vi "LEMP_realtime_theory_v3.vi"() -> ()   [LabVIEW 2021]
uses:
  <vilib>/Analysis/7linalg.llb/Eigenvalue and Vectors Output Option.ctl
  <vilib>/Analysis/baseanly.llb/Matrix Type of Inverse Matrix.ctl
  <vilib>/Analysis/4window.llb/Hanning Window (DBL).vi
  <vilib>/Analysis/5stat.llb/RMS (DBL).vi
  <vilib>/Analysis/4window.llb/Hamming Window (DBL).vi
  <vilib>/Analysis/2dsp.llb/Real FFT.vi
  <vilib>/Analysis/7linalg.llb/Real Generalized Eigenvalues and Vectors.vi
  <vilib>/Analysis/7linalg.llb/Real Cholesky Factorization.vi
  <vilib>/Analysis/4window.llb/AllCosWindow (DBL).vi
  <vilib>/Analysis/baseanly.llb/Full Cholesky Factorization.vi
  <vilib>/Analysis/baseanly.llb/Full Real Matrix Cholesky Factorization.vi
  <vilib>/addons/Time Series Analysis/Series Preprocess.llb/TSA Moving Average (Array).vi
  <vilib>/Analysis/Matrix/Numeric/Conversions/Array To Matrix - RA2.vi
  <vilib>/Analysis/baseanly.llb/Real Inverse Matrix.vi
  <vilib>/Analysis/Matrix/Numeric/Multiply/Multiply - RM,RM.vi
  <vilib>/Analysis/7linalg.llb/Real Eigenvalues and Vectors.vi
  <vilib>/Analysis/Matrix/Numeric/Add/Add - RM,RM.vi
  <vilib>/gmath/statdist.llb/Normal Moments.vi
  <vilib>/gmath/NI_Gmath.lvlib
  <vilib>/Analysis/NI_AALPro.lvlib
  <vilib>/Analysis/Matrix/NI_Matrix.lvlib
  <vilib>/Analysis/NI_AALBase.lvlib
  <vilib>/DAQmx/write.llb/DAQmx Write (Digital 1D Bool NChan 1Samp 1Line).vi
  <vilib>/addons/_Advanced Signal Processing/NI_AdvSigProcTSA.lvlib
panel:
  in  "Modeling Parameters":T1
  in  "Sub Sample":bool
  out "min value":dbl=40.777955555555565
  out "max value":dbl=69.90506666666668
  in  "MASTER":bool
  in  "Tab Control":T2(tab)=enum."Check"
  out "Cycle time (ms)":dbl=0.147275536505731
  out "1st Nat. Freq. (Hz) 2":dbl=40.777955555555565 format="%#_5g"
  out "FEA Frequencies":dbl[](array[numeric])=[47.056894447356875, 51.47067845292848, 50.76081786160022]
  out "Acceleration Data":dbl[](graph) caption="Accelorometer data"
  in  "Real-Time plotting":bool
  out "Probability Density Function":cluster{i32[], dbl[]}(graph)={[9, 10, 11, 12, 13, 14, 15, 16, 17, 18, 19, 20, 21, 22, 23, 24, 25, 26], [0.09171563397251428, 0.12108231855717679, 0.143041857841436, 0.1512135165862316, 0.143041857841436, 0.12108231855717679, 0.09171563397251428, 0.062165735159412254, 0.03770542435775916, 0.020464524096401888, 0.009939041952144324, 0.004319489826678621, 0.0016798304322918924, 0.0005845793791312176, 0.00018203990329545533, 5.072648364839732e-05, 1.2648760741233286e-05, 2.8223200098705454e-06]}
  out "FFT":dbl[](graph)
  out "Frequencies":dynamicdata(graph)=[{"t0"=timestamp(0 s since 1904-01-01), "dt"=1.0, "Y"=array[322 elements]}, {"t0"=timestamp(0 s since 1904-01-01), "dt"=1.0, "Y"=array[322 elements]}]
  out "Position":dynamicdata(graph)=[{"t0"=timestamp(0 s since 1904-01-01), "dt"=1.0, "Y"=[10.0, 12.0, 10.0, 10.0, 10.0, 9.0, 10.0, 12.0, 10.0, 9.0, 9.0, 12.0, 10.0, 16.0, 11.0, 14.0, 14.0, 12.0, 12.0, 12.0, 12.0, 14.0, 14.0, 11.0, 12.0, 12.0, 12.0, 12.0, 12.0, 10.0, 12.0, 14.0, 13.0, 16.0, 14.0, 13.0, 16.0, 14.0, 11.0, 11.0, 16.0, 18.0, 11.0, 10.0, 10.0, 12.0, 10.0, 10.0, 12.0, 12.0, 10.0, 12.0, 10.0, 10.0, 10.0, 10.0, 12.0, 9.0, 11.0, 13.0, 15.0, 15.0, 16.0, 18.0, 15.0, 15.0, 17.0, 15.0, 20.0, 18.0, 15.0, 15.0, 11.0, 11.0, 11.0, 12.0, 9.0, 10.0, 10.0, 10.0, 10.0, 12.0, 14.0, 10.0, 12.0, 12.0, 10.0, 10.0, 10.0, 10.0, 10.0, 10.0, 9.0, 10.0, 12.0, 9.0, 9.0, 14.0, 11.0, 13.0, 15.0, 19.0, 19.0, 17.0, 17.0, 17.0, 21.0, 19.0, 26.0, 26.0, 26.0, 26.0, 24.0, 26.0, 24.0, 24.0, 21.0, 20.0, 20.0, 20.0, 22.0, 14.0, 16.0, 18.0, 18.0, 12.0, 10.0, 12.0, 12.0, 12.0, 16.0, 14.0, 10.0, 14.0, 16.0, 16.0, 20.0, 20.0, 22.0, 22.0, 26.0, 21.0, 19.0, 19.0, 15.0, 19.0, 19.0, 19.0, 19.0, 17.0, 20.0, 24.0, 23.0, 21.0, 21.0, 26.0, 26.0, 26.0, 26.0, 24.0, 24.0, 22.0, 20.0, 22.0, 24.0, 22.0, 24.0, 20.0, 17.0, 18.0, 16.0, 13.0, 14.0, 14.0, 12.0, 10.0, 9.0, 10.0, 11.0, 17.0, 17.0, 24.0, 21.0, 23.0, 24.0, 19.0, 21.0, 25.0, 23.0, 26.0, 25.0, 25.0, 23.0, 23.0, 21.0, 23.0, 25.0, 21.0, 26.0, 24.0, 22.0, 18.0, 14.0, 12.0, 12.0, 12.0, 10.0, 12.0, 10.0, 9.0, 10.0, 10.0, 12.0, 11.0, 10.0, 12.0, 10.0, 10.0, 10.0, 10.0, 10.0, 10.0, 10.0, 9.0, 12.0, 12.0, 11.0, 13.0, 14.0, 12.0, 12.0, 12.0, 10.0, 10.0, 12.0, 10.0, 10.0, 10.0, 9.0, 9.0, 10.0, 12.0, 12.0, 18.0, 14.0, 18.0, 15.0, 12.0, 12.0, 12.0, 14.0, 11.0, 12.0, 12.0, 12.0, 11.0, 10.0, 10.0, 9.0, 10.0, 14.0, 16.0, 12.0, 12.0, 13.0, 13.0, 15.0, 13.0, 14.0, 9.0, 9.0, 10.0, 10.0, 9.0, 10.0, 11.0, 10.0, 10.0, 12.0, 11.0, 14.0, 14.0, 12.0, 12.0, 10.0, 13.0, 15.0, 13.0, 15.0, 15.0, 21.0, 19.0, 16.0, 16.0, 14.0, 16.0, 14.0, 12.0, 10.0, 10.0, 10.0, 10.0, 14.0, 22.0, 24.0, 22.0, 26.0, 22.0, 20.0, 20.0, 19.0, 21.0, 21.0, 17.0, 19.0, 17.0, 16.0, 17.0, 14.0, 12.0, 12.0, 10.0]}, {"t0"=timestamp(0 s since 1904-01-01), "dt"=1.0, "Y"=[9.0, 9.0, 9.0, 10.0, 11.0, 11.0, 12.0, 12.0, 12.0, 12.0, 11.0, 11.0, 10.0, 10.0, 9.0, 9.0, 9.0, 9.0, 10.0, 10.0, 11.0, 11.0, 11.0, 12.0, 12.0, 13.0, 13.0, 14.0, 14.0, 14.0, 14.0, 14.0, 15.0, 15.0, 15.0, 14.0, 13.0, 13.0, 12.0, 11.0, 10.0, 10.0, 10.0, 9.0, 9.0, 9.0, 9.0, 9.0, 10.0, 11.0, 11.0, 12.0, 12.0, 13.0, 14.0, 15.0, 16.0, 16.0, 16.0, 17.0, 17.0, 17.0, 17.0, 17.0, 17.0, 17.0, 16.0, 16.0, 15.0, 15.0, 14.0, 13.0, 12.0, 11.0, 11.0, 10.0, 10.0, 10.0, 9.0, 9.0, 9.0, 9.0, 9.0, 9.0, 9.0, 10.0, 11.0, 12.0, 12.0, 13.0, 14.0, 14.0, 15.0, 15.0, 16.0, 17.0, 18.0, 19.0, 19.0, 19.0, 20.0, 20.0, 20.0, 20.0, 20.0, 19.0, 19.0, 19.0, 18.0, 18.0, 17.0, 16.0, 15.0, 15.0, 14.0, 13.0, 12.0, 11.0, 11.0, 10.0, 10.0, 10.0, 9.0, 9.0, 9.0, 9.0, 9.0, 10.0, 10.0, 11.0, 12.0, 13.0, 14.0, 15.0, 16.0, 18.0, 19.0, 20.0, 21.0, 21.0, 22.0, 22.0, 22.0, 23.0, 23.0, 23.0, 23.0, 23.0, 22.0, 22.0, 22.0, 21.0, 21.0, 20.0, 19.0, 18.0, 16.0, 15.0, 14.0, 13.0, 12.0, 12.0, 12.0, 11.0, 10.0, 10.0, 9.0, 9.0, 9.0, 9.0, 10.0, 10.0, 11.0, 12.0, 13.0, 15.0, 16.0, 18.0, 20.0, 21.0, 22.0, 23.0, 24.0, 25.0, 25.0, 25.0, 25.0, 25.0, 25.0, 25.0, 24.0, 23.0, 22.0, 21.0, 20.0, 19.0, 17.0, 15.0, 14.0, 13.0, 12.0, 11.0, 10.0, 10.0, 9.0, 9.0, 9.0, 9.0, 9.0, 9.0, 9.0, 9.0, 9.0, 9.0, 9.0, 9.0, 9.0, 10.0, 11.0, 11.0, 10.0, 9.0, 9.0, 9.0, 9.0, 9.0, 9.0, 9.0, 9.0, 9.0, 9.0, 9.0, 9.0, 9.0, 9.0, 9.0, 9.0, 9.0, 9.0, 9.0, 10.0, 13.0, 14.0, 13.0, 11.0, 10.0, 9.0, 9.0, 9.0, 9.0, 9.0, 9.0, 9.0, 9.0, 9.0, 9.0, 9.0, 9.0, 9.0, 9.0, 9.0, 10.0, 14.0, 16.0, 17.0, 14.0, 12.0, 10.0, 9.0, 9.0, 9.0, 9.0, 9.0, 9.0, 9.0, 9.0, 9.0, 9.0, 9.0, 9.0, 9.0, 9.0, 10.0, 14.0, 18.0, 19.0, 20.0, 18.0, 14.0, 10.0, 9.0, 9.0, 9.0, 9.0, 9.0, 9.0, 9.0, 9.0, 9.0, 9.0, 9.0, 9.0, 9.0, 9.0, 9.0, 10.0, 13.0, 18.0, 22.0, 22.0, 19.0, 15.0, 12.0, 10.0, 9.0, 9.0, 9.0, 9.0, 9.0, 9.0, 9.0, 9.0]}]
  in  "PDF":bool
  out "Low-Energy Warning":bool
  in  "Frequency Method":T3(ring)=enum."1-FFT-CPU"
  in  "Width":dbl=0.0508 format="%#.6f"
  in  "Density":dbl=7900.0
  in  "Height":dbl=0.00635
  in  "Length of Beam":dbl=0.3525
  in  "Young's Modulus":dbl=209500000000.0
  in  "Torsion Spring":dbl format="%#.6f"
  in  "Initial Pin node":i32
  in  "Std. Dev.":dbl=0.5 min=0.0
  in  "Eigenvalue Method":T4(ring)
  out "average cycle time (ms)":dbl=4.283940110367686 format="%0.2f"
  in  "FFT data length (data points)":i32=15000
  in  "Min. FFT Power Value (RMS)":dbl=0.02
  in  "Bound to 1st Frequency":bool=TRUE
  in  "accelerometer_mass":dbl=0.055
  in  "Std. Dev = Number of Particles / 3":bool=TRUE
  out "Std. Dev.  2":dbl=1.0
  in  "Number Of Particles":i32=3
  in  "FEA Nodes":i32=60
  in  "file name":i32
  out "FFT_data_length":i32=15000
  in  "Auto FFT length":bool
  out "Hz / per pin location":dbl=1.0
  out "FFT_frequency_resolution":dbl=1.7066666666666668
  in  "scaling_factor_Hz_per_pin_to_frequency_resolution":dbl=0.33 caption="Scale FFT Factor" format="%#_13g"
  in  "Save Acceleration Data":bool=TRUE
  in  "Mode Count":i32=3 min=1 max=10 step=1
  in  "Max Roller Velocity":dbl=3.32
  in  "Frequency selection method":T5(ring)
  in  "Use Top N freq components":i32=5 min=1 max=50 step=1
  out "Std. Dev. 2":dbl=1.0
  out "1st Nat. Freq. (Hz) 4":waveform(dbl)[](graph)=[{"t0"=timestamp(0 s since 1904-01-01), "dt"=0.004283940110367686, "Y"=array[2994 elements]}, {"t0"=timestamp(0 s since 1904-01-01), "dt"=0.004283940110367686, "Y"=array[2994 elements]}] caption="1st Nat. Freq. (Hz)"
  out "1st Nat. Freq. (Hz) 5":waveform(dbl)[](graph)=[{"t0"=timestamp(0 s since 1904-01-01), "dt"=0.004283940110367686, "Y"=array[2994 elements]}, {"t0"=timestamp(0 s since 1904-01-01), "dt"=0.004283940110367686, "Y"=array[2994 elements]}] caption="Beam Boundary condtion"
  # "Note: All Inputs are based on base SI units."
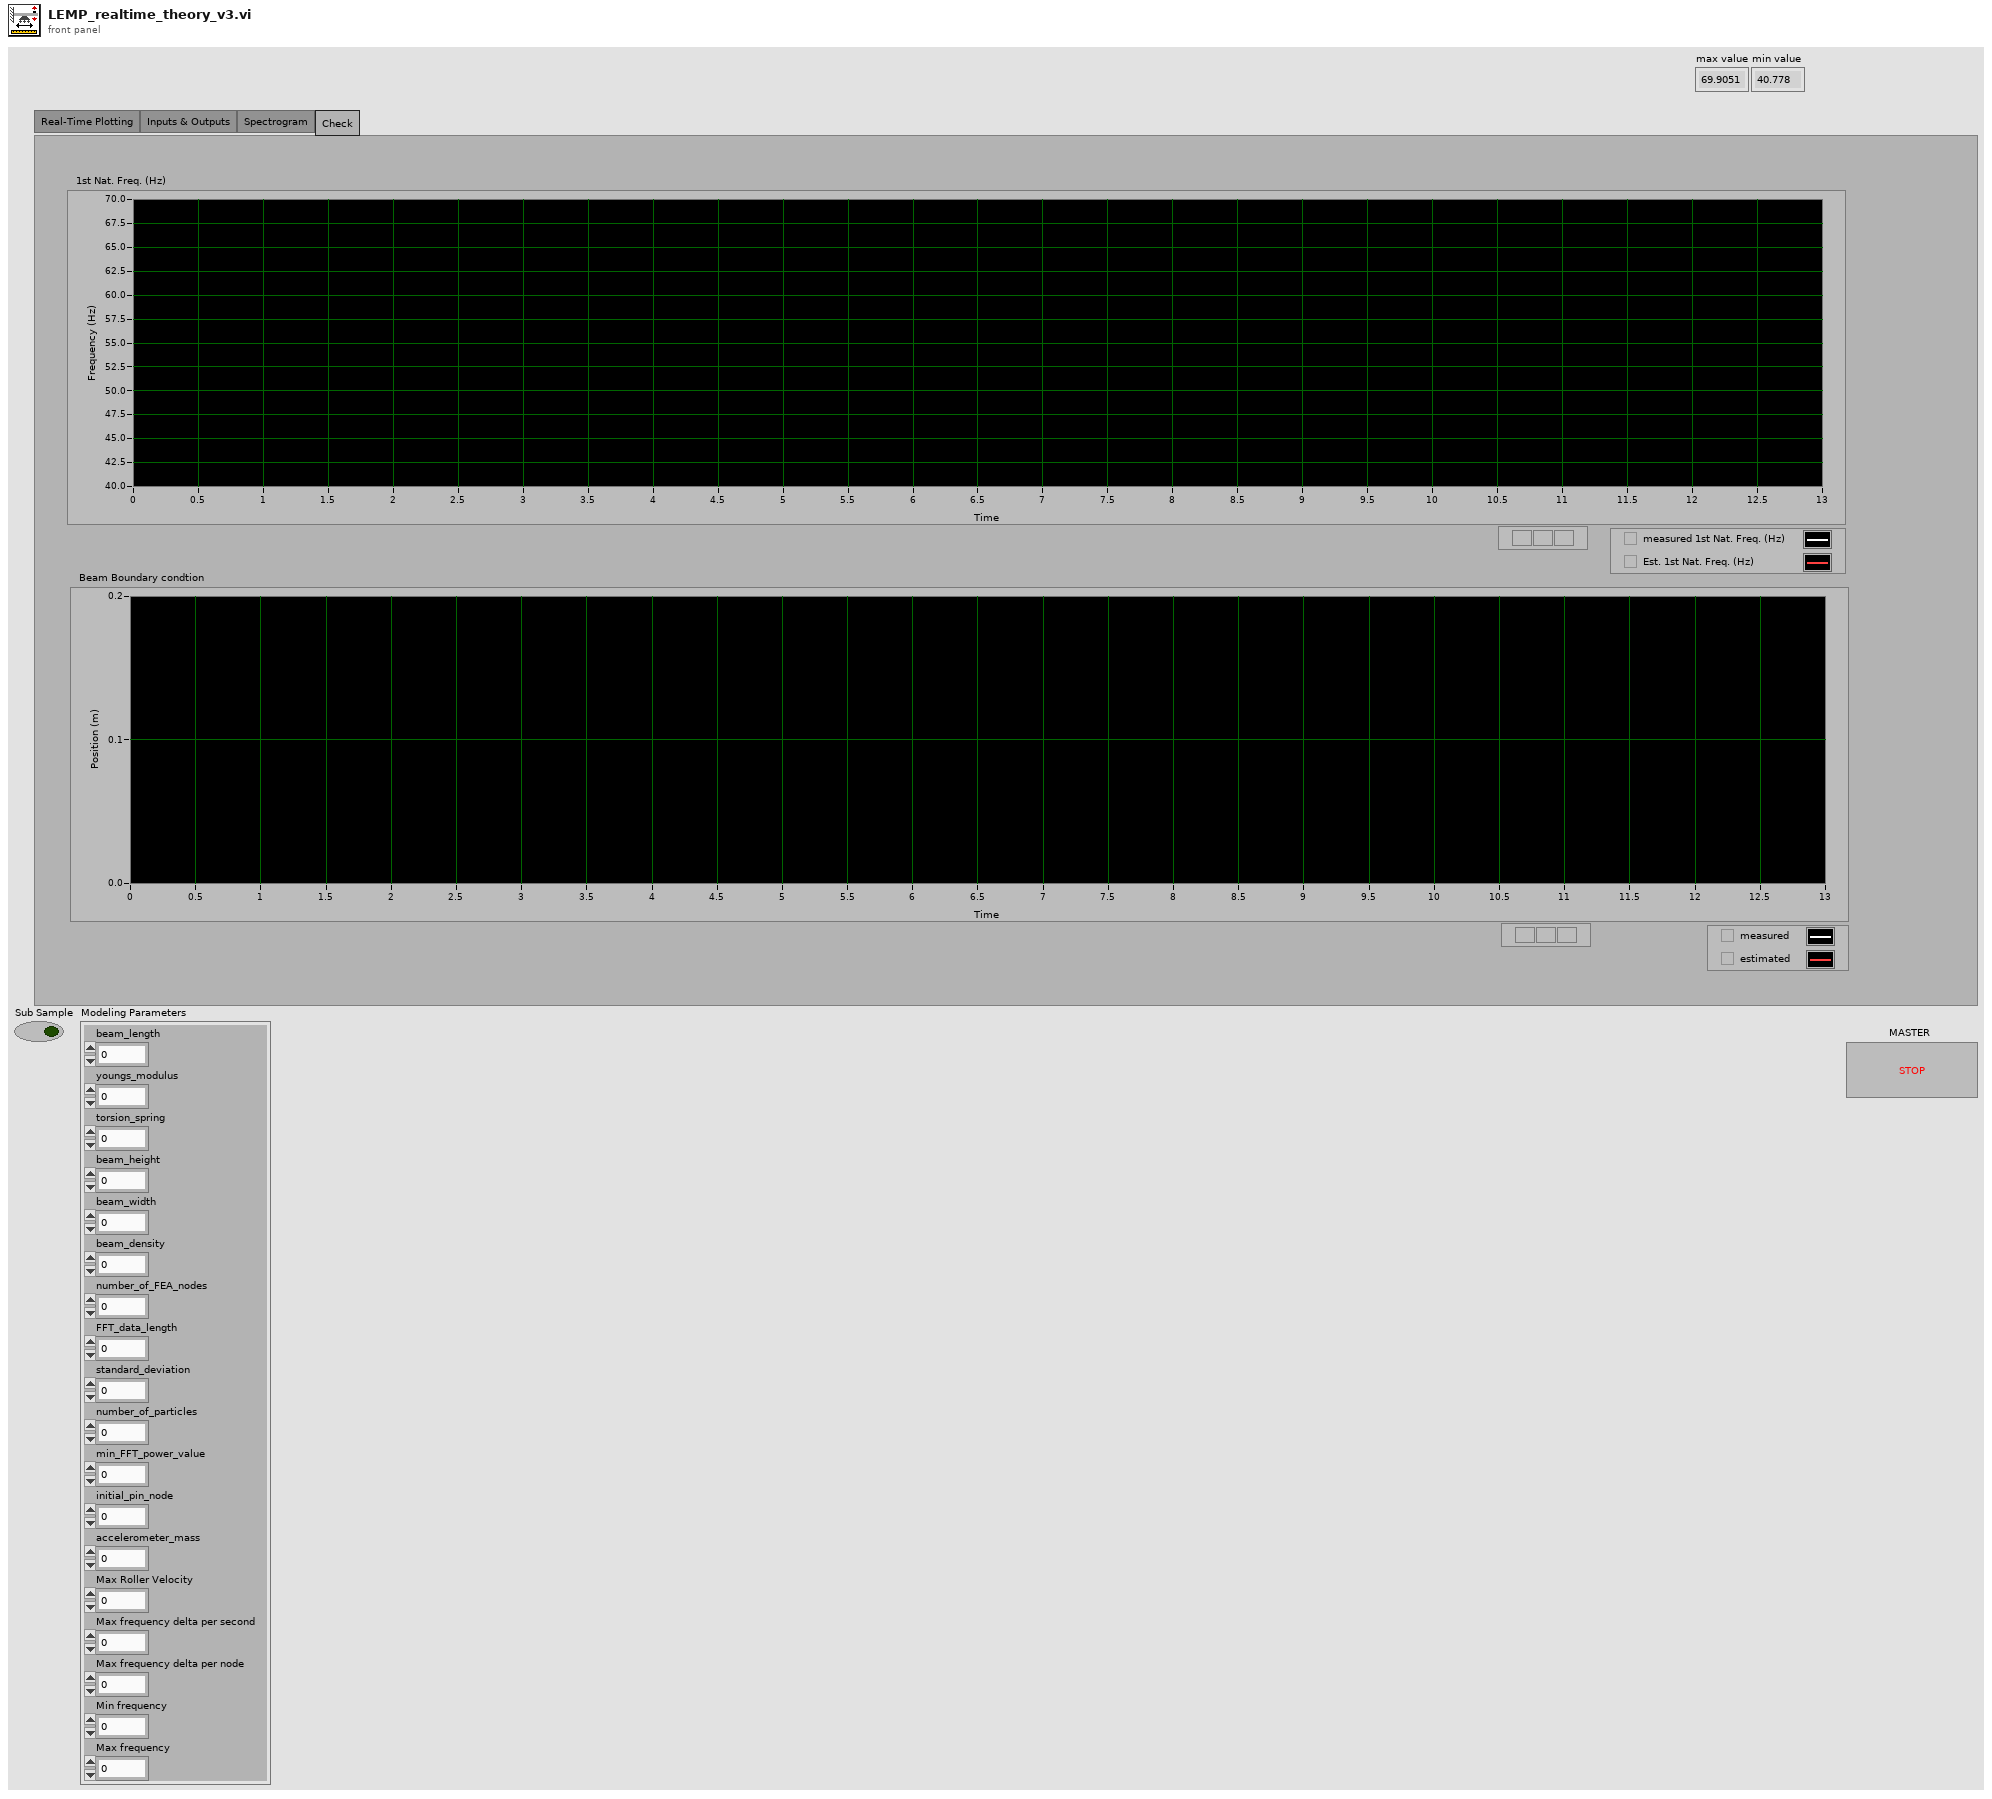
[diagram p1: front panel]
types:
  T1 = cluster{"beam_length":dbl, "youngs_modulus":dbl, "torsion_spring":dbl, "beam_height":dbl, "beam_width":dbl, "beam_density":dbl, "number_of_FEA_nodes":i32, "FFT_data_length":i32, "standard_deviation":dbl, "number_of_particles":i32, "min_FFT_power_value":dbl, "initial_pin_node":i32, "accelerometer_mass":dbl, "Max Roller Velocity":dbl, "Max frequency delta per second":dbl, "Max frequency delta per node":dbl, "Min frequency":dbl, "Max frequency":dbl}
  T2 = enum32{"Real-Time Plotting", "Inputs & Outputs", "Spectrogram", "Check"}
  T3 = enum16{"0-Tone", "1-FFT-CPU", "2-Custom Filter", "3-Bandpass FFT"}
  T4 = enum16{"0-Local Eigen Modification Procedure", "1-LabVIEW generalized eigenvalues", "2-LabVIEW M^-1K eigenvalues", "3-LabVIEW Cholesky Factorization", "4-Cholesky Factorization CPU SGL", "5-Cholesky Factorization CPU FXP", "6-Cholesky Factorization FPGA SGL", "7-Cholesky Factorization FPGA SGL SCL"}
  T5 = enum16{"0-Nearest component to prior ", "1-Coerce maximum differential", "2-Average with nearest component", "3-Top by power", "4-Lowest major component", "5-Average with lowest component"}
  T6 = cluster{"LEMP":cluster{"Eigenvalues":dbl[], "Square Transpose Eigenvectors":dbl[][], "1/deltaStiff":dbl}, "nodes of interest":i32[], "all nodes":i32[], "Eigenvalue Method":enum16{"0-Local Eigen Modification Procedure", "1-LabVIEW generalized eigenvalues", "2-LabVIEW M^-1K eigenvalues", "3-LabVIEW Cholesky Factorization", "4-Cholesky Factorization CPU SGL", "5-Cholesky Factorization CPU FXP", "6-Cholesky Factorization FPGA SGL", "7-Cholesky Factorization FPGA SGL SCL"}, "Mode Count":i32, "initial_pin_node":i32, "Sub Sample":bool}
  T7 = cluster{"beam_length":dbl, "youngs_modulus":dbl, "torsion_spring":dbl, "beam_height":dbl, "beam_width":dbl, "beam_density":dbl, "number_of_FEA_nodes":i32, "FFT_data_length":i32, "standard_deviation":dbl, "number_of_particles":i32, "min_FFT_power_value":dbl, "initial_pin_node":i32, "accelerometer_mass":dbl}
  T8 = cluster{"time_average_cycle":dbl, "measured_frequency":dbl[], "date_time":string, "estimated_pin_node":i32[], "time_cycle_start":dbl[], "measured_pin_location":dbl[], "estimated_frequency":dbl[], "acceleration_data":dbl[], "accelerometer_sample_rate":dbl, "displacement_sample_rate":dbl, "time_compare_start":dbl[], "time_subsample_start":dbl[], "time_FEA_start":dbl[], "time_FEA_end":dbl[], "time_cycle_end":dbl[], "time_accelerometer_aquire_start":dbl[], "time_frequency_calculations_start":dbl[], "time_frequency_calculations_end":dbl[], "measured_pin_location_tt":dbl[], "time_ACC_data_collection_start":dbl, "time_acceleration_data":dbl[], "estimated_pin_location":dbl[], "scaling_factor_Hz_per_pin_to_frequency_resolution":dbl, "Std_Dev_equale_particles_divided_3":bool, "Auto_FFT_length":bool, "windowed_acc_data":dbl[][], "FFT":dbl[][]}
  T9 = cluster{"Experimental Replay":cluster{"Accelorometer":dbl[], "Displacement":dbl[], "dt":dbl, "Final Time":dbl}, "Experimental Results":cluster{"time_average_cycle":dbl, "measured_frequency":dbl[], "date_time":string, "estimated_pin_node":i32[], "time_cycle_start":dbl[], "measured_pin_location":dbl[], "estimated_frequency":dbl[], "acceleration_data":dbl[], "accelerometer_sample_rate":dbl, "displacement_sample_rate":dbl, "time_compare_start":dbl[], "time_subsample_start":dbl[], "time_FEA_start":dbl[], "time_FEA_end":dbl[], "time_cycle_end":dbl[], "time_accelerometer_aquire_start":dbl[], "time_frequency_calculations_start":dbl[], "time_frequency_calculations_end":dbl[], "measured_pin_location_tt":dbl[], "time_ACC_data_collection_start":dbl, "time_acceleration_data":dbl[], "estimated_pin_location":dbl[], "scaling_factor_Hz_per_pin_to_frequency_resolution":dbl, "Std_Dev_equale_particles_divided_3":bool, "Auto_FFT_length":bool, "windowed_acc_data":dbl[][], "FFT":dbl[][]}, "FEA Parameters":cluster{"LEMP":cluster{"Eigenvalues":dbl[], "Square Transpose Eigenvectors":dbl[][], "1/deltaStiff":dbl}, "nodes of interest":i32[], "all nodes":i32[], "Eigenvalue Method":enum16{"0-Local Eigen Modification Procedure", "1-LabVIEW generalized eigenvalues", "2-LabVIEW M^-1K eigenvalues", "3-LabVIEW Cholesky Factorization", "4-Cholesky Factorization CPU SGL", "5-Cholesky Factorization CPU FXP", "6-Cholesky Factorization FPGA SGL", "7-Cholesky Factorization FPGA SGL SCL"}, "Mode Count":i32, "initial_pin_node":i32, "Sub Sample":bool}, "Modeling Parameters":cluster{"beam_length":dbl, "youngs_modulus":dbl, "torsion_spring":dbl, "beam_height":dbl, "beam_width":dbl, "beam_density":dbl, "number_of_FEA_nodes":i32, "FFT_data_length":i32, "standard_deviation":dbl, "number_of_particles":i32, "min_FFT_power_value":dbl, "initial_pin_node":i32, "accelerometer_mass":dbl, "Max Roller Velocity":dbl, "Max frequency delta per second":dbl, "Max frequency delta per node":dbl, "Min frequency":dbl, "Max frequency":dbl}}
  T10 = cluster{"Accelorometer":dbl[], "Displacement":dbl[], "dt":dbl, "Final Time":dbl}
  T11 = typedef "NI_AALBase.lvlib/Matrix Type of Inverse Matrix.ctl" = enum32{"General", "Positive Definite", "Lower Triangular", "Upper Triangular"}
  T12 = cluster{"Eigenvalues":dbl[], "Square Transpose Eigenvectors":dbl[][], "1/deltaStiff":dbl}
  T13 = typedef "NI_AALPro.lvlib/Eigenvalue and Vectors Output Option.ctl" = i32
  T14 = typedef "NI_Matrix.lvlib/RealMatrix.ctl" = dbl[][]
  T15 = cluster{"nodes of interest":i32[], "Sample PDF":dbl[]}
  T16 = cluster{"time_average_cycle":dbl, "measured_frequency":dbl[], "date_time":string, "estimated_pin_node":i32[], "time_cycle_start":dbl[], "measured_pin_location":dbl[], "estimated_frequency":dbl[], "acceleration_data":dbl[], "accelerometer_sample_rate":dbl, "displacement_sample_rate":dbl, "time_compare_start":dbl[], "time_subsample_start":dbl[], "time_FEA_start":dbl[], "time_FEA_end":dbl[], "time_cycle_end":dbl[], "time_accelerometer_aquire_start":dbl[], "time_frequency_calculations_start":dbl[], "time_frequency_calculations_end":dbl[], "measured_pin_location_tt":dbl[], "time_ACC_data_collection_start":dbl, "time_acceleration_data":dbl[], "estimated_pin_location":dbl[], "scaling_factor_Hz_per_pin_to_frequency_resolution":dbl, "Std_Dev_equale_particles_divided_3":bool, "Auto_FFT_length":bool, "windowed_acc_data":dbl[][], "FFT":dbl[][], "beam_length":dbl, "youngs_modulus":dbl, "torsion_spring":dbl, "beam_height":dbl, "beam_width":dbl, "beam_density":dbl, "number_of_FEA_nodes":i32, "FFT_data_length":i32, "standard_deviation":dbl, "number_of_particles":i32, "min_FFT_power_value":dbl, "initial_pin_node":i32, "accelerometer_mass":dbl}
  T17 = cluster{"measured_pin_location_tt":dbl[], "measured_pin_location":dbl[]}
  T18 = cluster{"time_acceleration_data":dbl[], "acceleration_data":dbl[]}
  T19 = cluster{"time_cycle_end":dbl[], "estimated_pin_location":dbl[]}
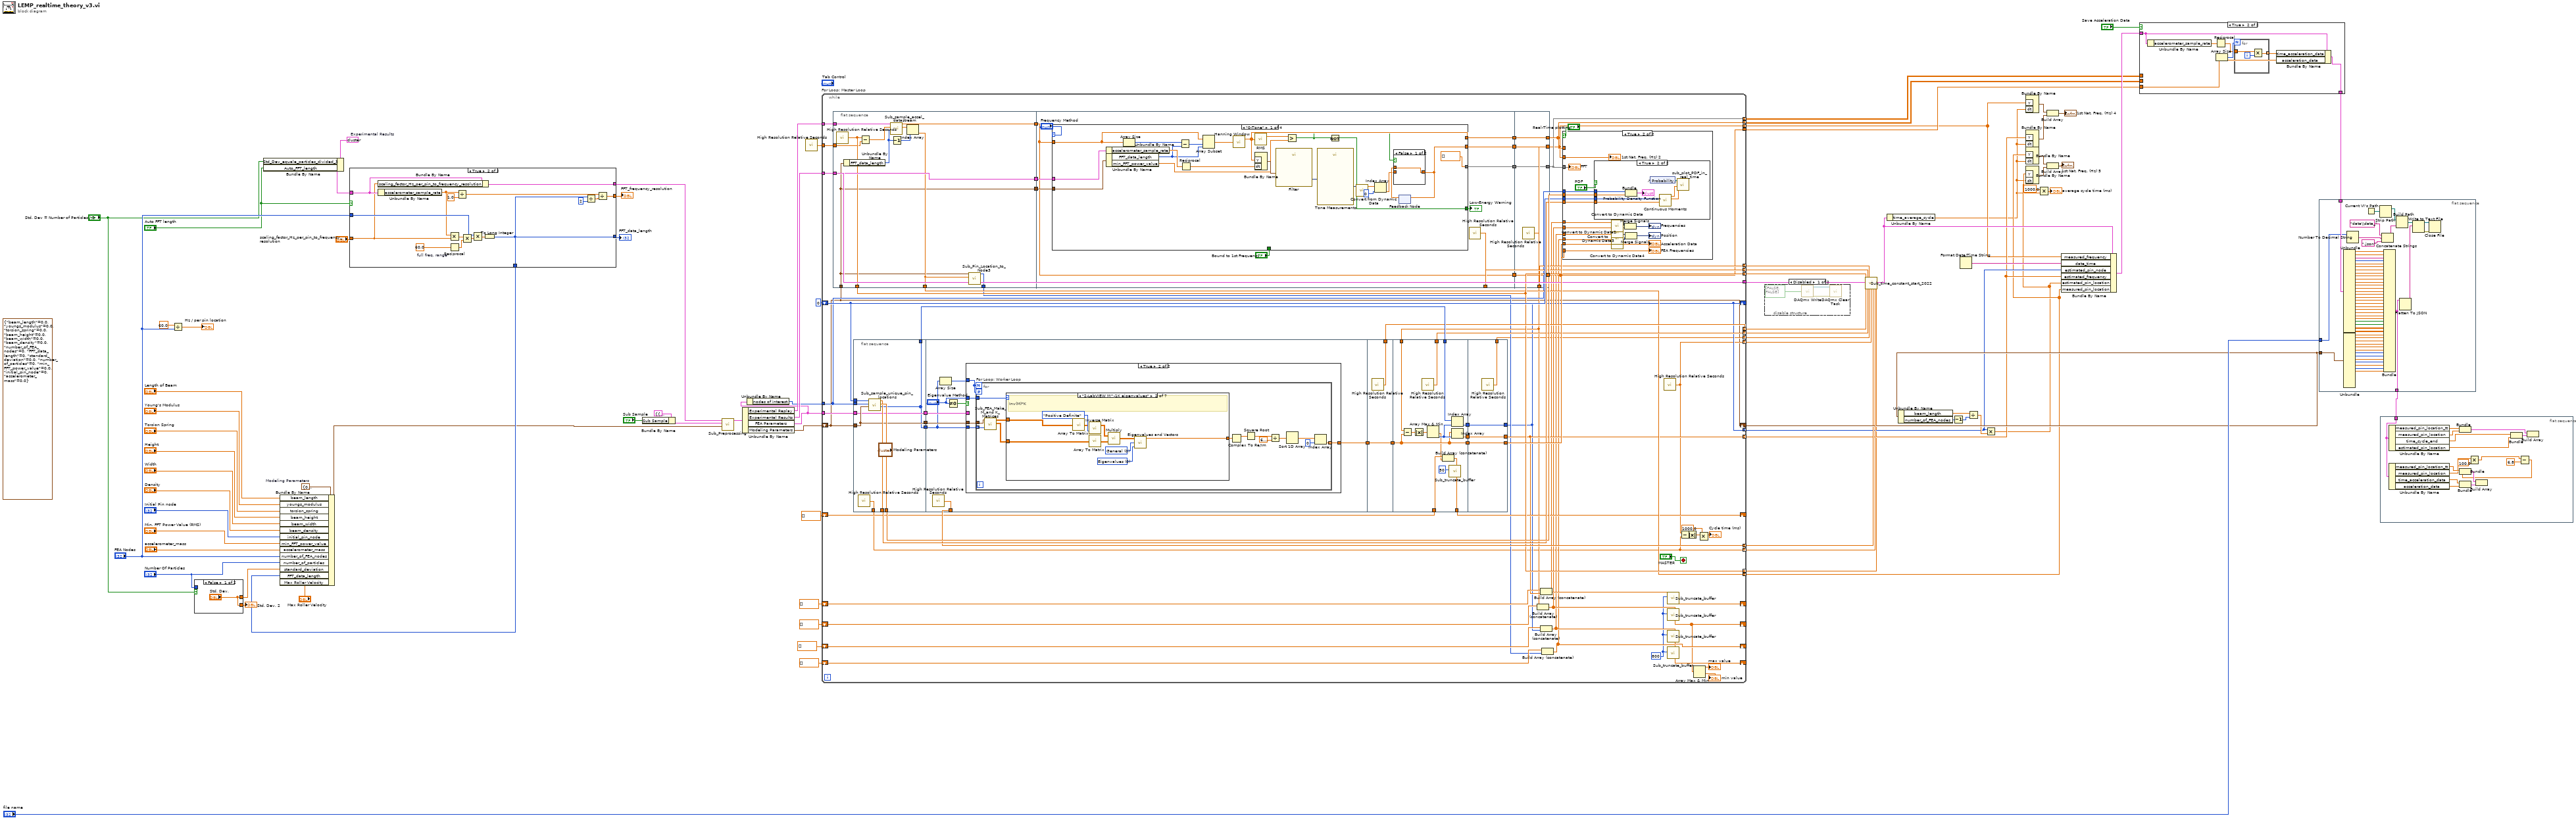
[diagram p0: block diagram]
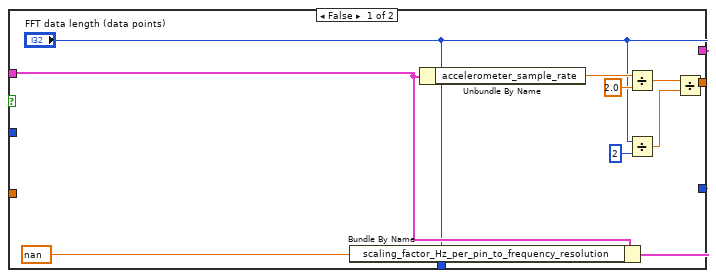
[diagram p4: hidden frame]
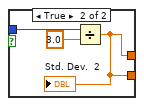
[diagram p5: hidden frame]
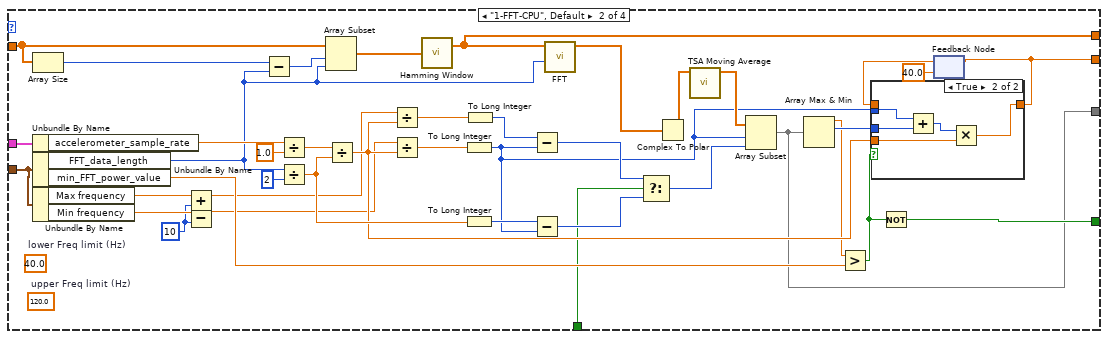
[diagram p7: hidden frame]
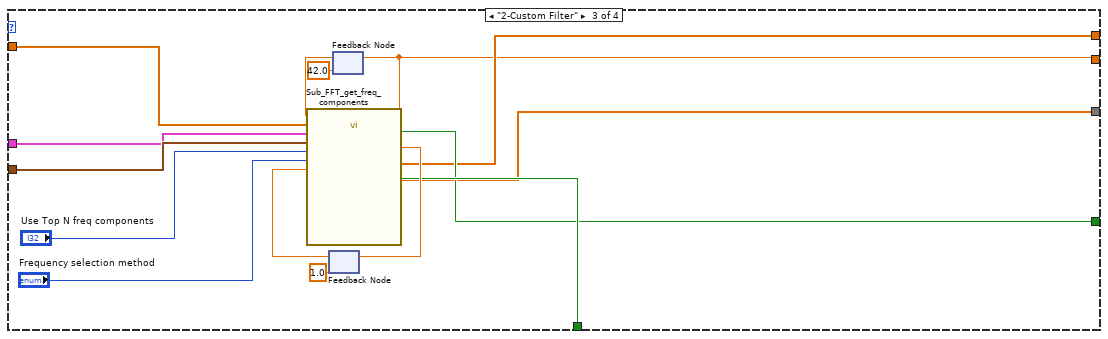
[diagram p9: hidden frame]
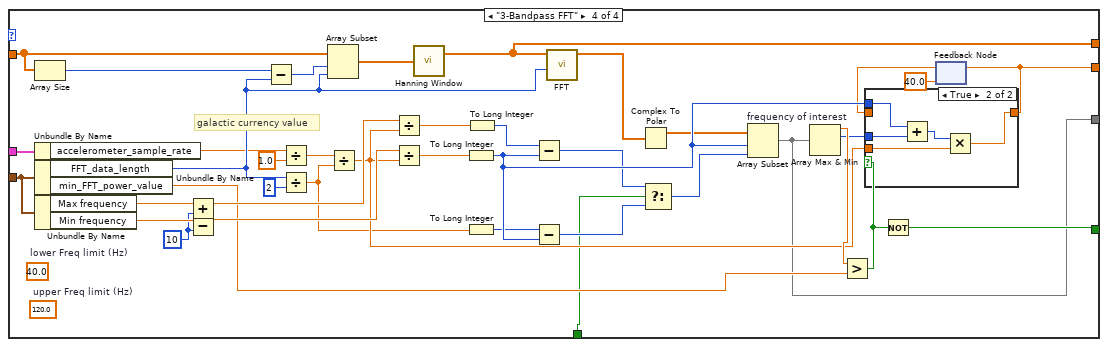
[diagram p10: hidden frame]
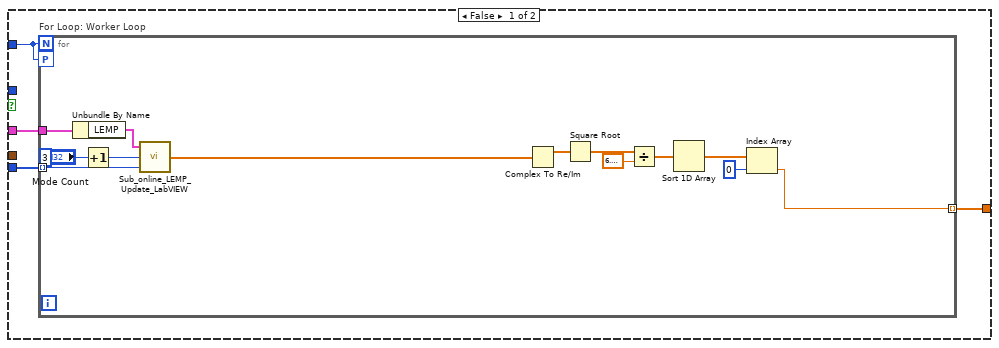
[diagram p12: hidden frame]
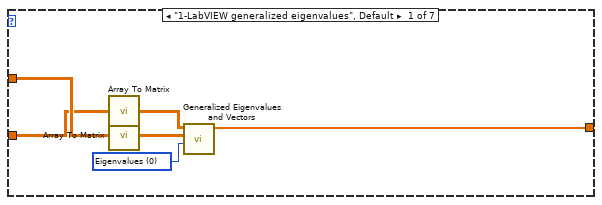
[diagram p13: hidden frame]
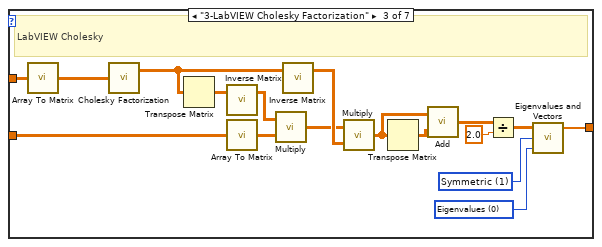
[diagram p14: hidden frame]
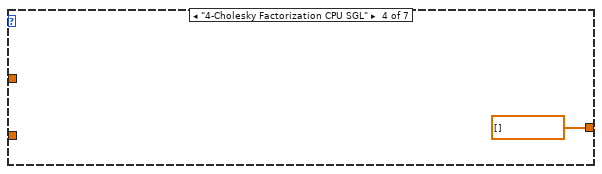
[diagram p15: hidden frame]
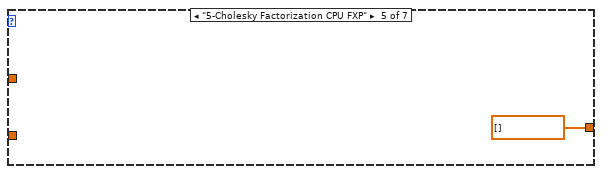
[diagram p16: hidden frame]
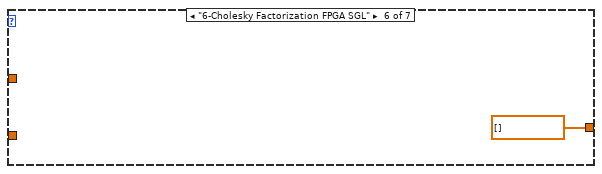
[diagram p17: hidden frame]
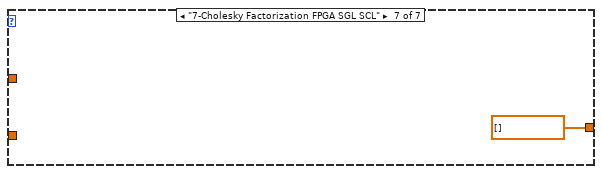
[diagram p18: hidden frame]
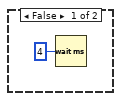
[diagram p20: hidden frame]
diagram:
  w11 = T1 {"beam_length"=0.0, "youngs_modulus"=0.0, "torsion_spring"=0.0, "beam_height"=0.0, "beam_width"=0.0, "beam_density"=0.0, "number_of_FEA_nodes"=0, "FFT_data_length"=0, "standard_deviation"=0.0, "number_of_particles"=0, "min_FFT_power_value"=0.0, "initial_pin_node"=0, "accelerometer_mass"=0.0, "Max Roller Velocity"=0.0, "Max frequency delta per second"=0.0, "Max frequency delta per node"=0.0, "Min frequency"=0.0, "Max frequency"=0.0}  # Modeling Parameters
  (unwired) T7 {"beam_length"=0.0, "youngs_modulus"=0.0, "torsion_spring"=0.0, "beam_height"=0.0, "beam_width"=0.0, "beam_density"=0.0, "number_of_FEA_nodes"=0, "FFT_data_length"=0, "standard_deviation"=0.0, "number_of_particles"=0, "min_FFT_power_value"=0.0, "initial_pin_node"=0, "accelerometer_mass"=0.0} ("Setup Parameters")
  w56 = T8 {"time_average_cycle"=0.0, "measured_frequency"=[], "date_time"="", "estimated_pin_node"=[], "time_cycle_start"=[], "measured_pin_location"=[], "estimated_frequency"=[], "acceleration_data"=[], "accelerometer_sample_rate"=0.0, "displacement_sample_rate"=0.0, "time_compare_start"=array[564 elements], "time_subsample_start"=array[564 elements], "time_FEA_start"=array[564 elements], "time_FEA_end"=array[564 elements], "time_cycle_end"=array[564 elements], "time_accelerometer_aquire_start"=array[564 elements], "time_frequency_calculations_start"=array[564 elements], "time_frequency_calculations_end"=array[564 elements], "measured_pin_location_tt"=array[564 elements], "time_ACC_data_collection_start"=0.0, "time_acceleration_data"=array[564 elements], "estimated_pin_location"=array[564 elements], "scaling_factor_Hz_per_pin_to_frequency_resolution"=1.0, "Std_Dev_equale_particles_divided_3"=TRUE, "Auto_FFT_length"=TRUE, "windowed_acc_data"=array1x564[564 elements], "FFT"=array1x564[564 elements]}  # Experimental Results
  n1 = Divide(x=60.0, y="FEA Nodes") -> (x/y=→"Hz / per pin location":dbl)
  n2 = case shown="False" "Std. Dev = Number of Particles / 3" {
    tunnel: ["Std. Dev." w85] -> w41
    tunnel: "Number Of Particles" -> [_ w86]
    tunnel: ["Std. Dev." w85] -> w83
    frame False {
    }
    frame True {
      n3 = Divide(x=w86, y=3.0) -> (x/y=w85:dbl)
      "Std. Dev.  2" <- w85
    }
  }
  "Std. Dev. 2" <- w83
  n4 = Bundle By Name(cluster=w56, "Std_Dev_equale_particles_divided_3"="Std. Dev = Number of Particles / 3", "Auto_FFT_length"="Auto FFT length") -> (w17:T8)
  n5 = case shown="True" "Auto FFT length" {
    tunnel: "FEA Nodes" -> [_ w105]
    tunnel: w17 -> [w91 w102]
    tunnel: ["FFT data length (data points)" w100] -> w42
    tunnel: [w92 w104] -> w55
    tunnel: ["FFT data length (data points)" w100] -> w54
    tunnel: [w90 w101] -> w10
    tunnel: "scaling_factor_Hz_per_pin_to_frequency_resolution" -> [_ w99]
    frame False {
      n6 = Bundle By Name(cluster=w91, "scaling_factor_Hz_per_pin_to_frequency_resolution"=nan) -> (w90:T8)
      n7 = Unbundle By Name(w91) -> ("accelerometer_sample_rate"=w97:dbl)
      n8 = Divide(x=w97, y=2.0) -> (x/y=w95:dbl)
      n9 = Divide(x="FFT data length (data points)", y=2) -> (x/y=w96:dbl)
      n10 = Divide(x=w95, y=w96) -> (x/y=w92:dbl)
    }
    frame True {
      w108 = 60.0  # full freq. range
      n11 = Bundle By Name(cluster=w102, "scaling_factor_Hz_per_pin_to_frequency_resolution"=w99) -> (w101:T8)
      n12 = Unbundle By Name(w102) -> ("accelerometer_sample_rate"=w98:dbl)
      n13 = Multiply(x=w98, y=w99) -> (x*y=w111:dbl)
      n14 = Reciprocal(x=w108) -> (1/x=w112:dbl)
      n15 = Divide(x=w98, y=1.0) -> (x/y=w109:dbl)
      n16 = Multiply(x=w111, y=w112) -> (x*y=w113:dbl)
      n17 = Multiply(x=w105, y=w113) -> (x*y=w103:dbl)
      n18 = To Long Integer(number=w103) -> (32bit integer=w100:i32)
      n19 = Divide(x=w100, y=2) -> (x/y=w110:dbl)
      n20 = Divide(x=w109, y=w110) -> (x/y=w104:dbl)
    }
  }
  "FFT_frequency_resolution" <- w55
  "FFT_data_length" <- w54
  n21 = Bundle By Name(cluster=w11, "beam_length"="Length of Beam", "youngs_modulus"="Young's Modulus", "torsion_spring"="Torsion Spring", "beam_height"="Height", "beam_width"="Width", "beam_density"="Density", "initial_pin_node"="Initial Pin node", "min_FFT_power_value"="Min. FFT Power Value (RMS)", "accelerometer_mass"="accelerometer_mass", "number_of_FEA_nodes"="FEA Nodes", "number_of_particles"="Number Of Particles", "standard_deviation"=w41, "FFT_data_length"=w42, "Max Roller Velocity"="Max Roller Velocity") -> (w12:T1)
  n22 = Bundle By Name(cluster=T6 {"LEMP"={"Eigenvalues"=[], "Square Transpose Eigenvectors"=[], "1/deltaStiff"=0.0}, "nodes of interest"=[], "all nodes"=[], "Eigenvalue Method"=enum."0-Local Eigen Modification Procedure", "Mode Count"=3, "initial_pin_node"=0, "Sub Sample"=TRUE} ("FEA Parameters"), "Sub Sample"="Sub Sample") -> (w8:T6)
  n23 = call "Sub_Preprocessing.vi"("Modeling Parameters"=w12, "FEA Parameters"=w8, "Experimental Results"=w10) -> ("Experiment"=w6:T9)  [unwired: 8 in]
  n24 = Unbundle By Name(w6) -> ("Experimental Replay"=w3:T10, "Experimental Results"=w4:T8, "FEA Parameters"=w2:T6, "Modeling Parameters"=w5:T1)
  n25 = Unbundle By Name(w2) -> ("nodes of interest"=w1:i32[])
  n26 = call <vilib>:"High Resolution Relative Seconds.vi"() -> ("relative seconds"=w14:dbl)
  n27 = while "For Loop: Master Loop" {
    shift-right: [w130] -> _
    shift-left: 0 -> [w173]
    tunnel: [w142] -> w34 mode=indexing
    tunnel: w1 -> [w146]
    tunnel: [w130] -> w35 mode=indexing
    tunnel: [w140] -> w21 mode=indexing
    tunnel: w4 -> [w177]
    tunnel: [w177] -> w63
    tunnel: [w128] -> w68 mode=indexing
    tunnel: [w163] -> w36 mode=indexing
    tunnel: [w162] -> w71 mode=indexing
    tunnel: [w152] -> w66 mode=indexing
    tunnel: [w161] -> w69 mode=indexing
    tunnel: [w160] -> w70 mode=indexing
    tunnel: [w126] -> w72 mode=indexing
    tunnel: [w157] -> w65 mode=indexing
    tunnel: [w129] -> w67 mode=indexing
    tunnel: [w155] -> w33 mode=indexing
    tunnel: [w145] -> w32 mode=indexing
    tunnel: w2 -> [w153]
    tunnel: [w151] -> w20 mode=indexing
    tunnel: [w152] -> w31 mode=indexing
    shift-right: [w147] -> _
    shift-left: dbl[] [] ("array") -> [w148]
    shift-right: [w114] -> w61
    shift-left: w5 -> [w114]
    shift-right: [w143] -> _
    shift-left: dbl[] [] ("array") -> [w144]
    shift-right: [w119] -> _
    shift-left: dbl[] [] ("array") -> [w141]
    shift-right: [w137] -> _
    shift-left: dbl[] [] ("array") -> [w135]
    shift-right: [w120] -> _
    shift-left: dbl[] [] ("array") -> [w136]
    tunnel: w14 -> [w118]
    tunnel: w3 -> [w117]
    tunnel: [w115] -> w48
    stop <- "MASTER" stop-if-true
    w131 = 800 ("samples")
    n28 = flat-sequence {
      tunnel: w114 -> [w180]
      tunnel: w177 -> [w191]
      tunnel: [w191] -> w171
      tunnel: [w185] -> w170
      tunnel: [w180] -> w169
      tunnel: [w189] -> w152
      tunnel: [w183] -> w151
      tunnel: [w190] -> w134
      tunnel: w118 -> [w188]
      tunnel: w117 -> [w186]
      tunnel: w171 -> [w199]
      tunnel: w170 -> [w192]
      tunnel: w169 -> [w198]
      tunnel: [w201] -> w165
      tunnel: [w197] -> w164
      tunnel: [w195] -> w161
      tunnel: [w193] -> w149
      tunnel: [w192] -> w116
      tunnel: [w334] -> w140
      tunnel: [w337] -> w155
      tunnel: w165 -> [w337]
      tunnel: w164 -> [w334]
      tunnel: [w336] -> w160
      tunnel: w149 -> [w335]
      tunnel: [w335] -> w145
      tunnel: w116 -> [w333]
      tunnel: [w333] -> w115
      frame #0 {
        n29 = call <vilib>:"High Resolution Relative Seconds.vi"() -> ("relative seconds"=w189:dbl)
        n30 = Unbundle By Name(w180) -> ("FFT_data_length"=w181:i32)
        n31 = Subtract(x=w189, y=w188) -> (x-y=w187:dbl)
        n32 = call "Sub_sample_accel_datastream.vi"("FFT data length"=w181, "Simulation Time"=w187, "Experimental Replay"=w186) -> ("Displacment sample"=w184:dbl[], "Accelerometer sample"=w185:dbl[])  [unwired: 7 in]
        n33 = Decrement(x=w181) -> (x-1=w182:i32)
        n34 = Index Array(array=w184, index=w182) -> (element=w183:dbl)
        n35 = call "Sub_Pin_Location_to_Node3.vi"("Pin Location"=w183, "Modeling Parameters"=w180) -> ("DOF of Interest"=w190:i32)  [unwired: 9 in]
      }
      frame #1 {
        n36 = case shown="\"0-Tone\"" "Frequency Method" {
          tunnel: [w212 w241 w275 w294] -> w197
          tunnel: [w214 w244 w278 w289] -> w201
          tunnel: w192 -> [w216 w247 w281 w297]
          tunnel: [w209 w243 w279 w296] -> w200
          tunnel: w198 -> [w205 w227 w283 w288]
          tunnel: w199 -> [w207 w246 w282 w298]
          tunnel: "Bound to 1st Frequency" -> [_ w245 w284 w295]
          tunnel: [dbl[] [] ("Real freq comp (out)") w236 w273 w291] -> w193
          frame "0-Tone" {
            n37 = Unbundle By Name(w207) -> ("accelerometer_sample_rate"=w206:dbl)
            n38 = Unbundle By Name(w205) -> ("FFT_data_length"=w203:i32, "min_FFT_power_value"=w204:dbl)
            n39 = Array Size(array=w216) -> (size(s)=w224:i32)
            n40 = Subtract(x=w224, y=w203) -> (x-y=w223:i32)
            n41 = Reciprocal(x=w206) -> (1/x=w208:dbl)
            n42 = Array Subset(array=w216, index=w223, length=w203) -> (w217:dbl[])
            n43 = call-poly <vilib>:"Hanning Window.vi"("X"=w217) -> ("Windowed X"=w214:dbl[])  [unwired: 1 out]
            n44 = Bundle By Name("Y"=w214, "dt"=w208) -> (w218:waveform(dbl))  [unwired: 1 in]
            n45 = call-poly <vilib>:"RMS.vi"("X"=w214) -> ("rms value"=w210:dbl)  [unwired: 1 out]
            n46 = call "Filter"("Signal"=w218) -> ("Filtered Signal"=w219:dynamicdata)  [unwired: 9 in, 1 out]
            n47 = Greater?(x=w210, y=w204) -> (0:w211:bool)
            n48 = call "Tone Measurements"("Signals"=w219) -> ("Frequency"=w220:dynamicdata)  [unwired: 9 in, 1 out]
            n49 = Not(x=w211) -> (.not. x?=w209:bool)
            n50 = call "Convert from Dynamic Data"("Dynamic Data Type"=w220) -> ("Array"=w221:dbl[])  [unwired: 3 in]
            n51 = Index Array(array=w221, index=0) -> (element=w213:dbl)
            n52 = feedback #1() -> (w215:dbl)  [unwired: 1 in]
            n53 = case shown="False" w211 {
              tunnel: [w225 w226] -> w212
              tunnel: w215 -> [w225 _]
              tunnel: w213 -> [_ w226]
              frame False {
              }
              frame True {
              }
            }
            n54 = feedback-in #1(w212) -> ()
          }
          frame "1-FFT-CPU", Default {
            w230 = 10
            (unwired) 120.0  # upper Freq limit (Hz)
            (unwired) 40.0  # lower Freq limit (Hz)
            n55 = Array Size(array=w247) -> (size(s)=w259:i32)
            n56 = Unbundle By Name(w246) -> ("accelerometer_sample_rate"=w248:dbl)
            n57 = Unbundle By Name(w227) -> ("FFT_data_length"=w229:i32, "min_FFT_power_value"=w249:dbl)
            n58 = Unbundle By Name(w227) -> ("Max frequency"=w232:dbl, "Min frequency"=w234:dbl)
            n59 = Add(x=w232, y=w230) -> (x+y=w231:dbl)
            n60 = Subtract(x=w234, y=w230) -> (x-y=w233:dbl)
            n61 = Subtract(x=w259, y=w229) -> (x-y=w258:i32)
            n62 = Divide(x=w248, y=1.0) -> (x/y=w261:dbl)
            n63 = Divide(x=w229, y=2) -> (x/y=w260:dbl)
            n64 = Array Subset(array=w247, index=w258, length=w229) -> (w257:dbl[])
            n65 = Divide(x=w261, y=w260) -> (x/y=w255:dbl)
            n66 = Divide(x=w231, y=w255) -> (x/y=w254:dbl)
            n67 = Divide(x=w233, y=w255) -> (x/y=w265:dbl)
            n68 = call-poly <vilib>:"Hamming Window.vi"("X"=w257) -> ("Windowed X"=w244:dbl[])  [unwired: 1 out]
            n69 = To Long Integer(number=w265) -> (32bit integer=w235:i32)
            n70 = To Long Integer(number=w260) -> (32bit integer=w263:i32)
            n71 = To Long Integer(number=w254) -> (32bit integer=w253:i32)
            n72 = Subtract(x=w253, y=w235) -> (x-y=w251:i32)
            n73 = Subtract(x=w263, y=w235) -> (x-y=w250:i32)
            n74 = call-poly <vilib>:"FFT.vi"("FFT size"=w229, "X"=w244) -> ("FFT {X}"=w242:cdb[])  [unwired: 8 in, 1 out]
            n75 = Select(t=w251, s=w245, f=w250) -> (s? t:f=w252:i32)
            n76 = Complex To Polar(r * e^(i*theta)=w242) -> (r=w238:dbl[])  [unwired: 1 out]
            n77 = call-poly <vilib>:"TSA Moving Average.vi"("Xt"=w238) -> ("Xt out"=w237:dbl[])  [unwired: 9 in, 1 out]
            n78 = Array Subset(array=w237, index=w235, length=w252) -> (w236:dbl[])
            n79 = Array Max & Min(array=w236) -> (max value=w228:dbl, max index (indices)=w264:i32)  [unwired: 2 out]
            n80 = Greater?(x=w228, y=w249) -> (0:w256:bool)
            n81 = Not(x=w256) -> (.not. x?=w243:bool)
            n82 = feedback #2(40.0) -> (w240:dbl)
            n83 = case shown="True" w256 {
              tunnel: w264 -> [_ w268]
              tunnel: w235 -> [_ w269]
              tunnel: w255 -> [_ w270]
              tunnel: [w267 w271] -> w241
              tunnel: w240 -> [w267 _]
              frame False {
              }
              frame True {
                n84 = Add(x=w269, y=w268) -> (x+y=w272:i32)
                n85 = Multiply(x=w272, y=w270) -> (x*y=w271:dbl)
              }
            }
            n86 = feedback-in #2(w241) -> ()
          }
          frame "2-Custom Filter" {
            n87 = feedback #3(1.0 ("Slop factor (Feed back)")) -> (w286:dbl)
            n88 = feedback #4(42.0) -> (w285:dbl)
            n89 = call "Sub_FFT_get_freq_components.vi"("Prior Frequency Estimate (Feed forward)"=w285, "ACC Signal"=w281, "Experimental Results"=w282, "Modeling Parameters"=w283, "Use Top N freq components"="Use Top N freq components", "Frequency selection method"="Frequency selection method", "Slop factor (Feed forward)"=w286, "Bound to 1st Frequency"=w284) -> ("Windowed X (out)"=w278:dbl[], "Real freq comp (out)"=w273:dbl[], "Next Frequency Estimate"=w275:dbl, "Low Energy"=w279:bool, "Slop factor (Feed back)"=w287:dbl)  [unwired: 15 in]
            n90 = feedback-in #3(w287) -> ()
            n91 = feedback-in #4(w275) -> ()
          }
          frame "3-Bandpass FFT" {
            w299 = 10
            (unwired) 120.0  # upper Freq limit (Hz)
            (unwired) 40.0  # lower Freq limit (Hz)
            # "galactic currency value"
            n92 = Array Size(array=w297) -> (size(s)=w308:i32)
            n93 = Unbundle By Name(w298) -> ("accelerometer_sample_rate"=w318:dbl)
            n94 = Unbundle By Name(w288) -> ("FFT_data_length"=w325:i32, "min_FFT_power_value"=w317:dbl)
            n95 = Unbundle By Name(w288) -> ("Max frequency"=w323:dbl, "Min frequency"=w321:dbl)
            n96 = Add(x=w323, y=w299) -> (x+y=w324:dbl)
            n97 = Subtract(x=w321, y=w299) -> (x-y=w322:dbl)
            n98 = Subtract(x=w308, y=w325) -> (x-y=w309:i32)
            n99 = Divide(x=w318, y=1.0) -> (x/y=w306:dbl)
            n100 = Divide(x=w325, y=2) -> (x/y=w307:dbl)
            n101 = Array Subset(array=w297, index=w309, length=w325) -> (w290:dbl[])
            n102 = Divide(x=w306, y=w307) -> (x/y=w311:dbl)
            n103 = Divide(x=w324, y=w311) -> (x/y=w312:dbl)
            n104 = Divide(x=w322, y=w311) -> (x/y=w303:dbl)
            n105 = call-poly <vilib>:"Hanning Window.vi"("X"=w290) -> ("Windowed X"=w289:dbl[])  [unwired: 1 out]
            n106 = To Long Integer(number=w303) -> (32bit integer=w320:i32)
            n107 = To Long Integer(number=w307) -> (32bit integer=w305:i32)
            n108 = To Long Integer(number=w312) -> (32bit integer=w313:i32)
            n109 = Subtract(x=w313, y=w320) -> (x-y=w315:i32)
            n110 = Subtract(x=w305, y=w320) -> (x-y=w316:i32)
            n111 = call-poly <vilib>:"FFT.vi"("FFT size"=w325, "X"=w289) -> ("FFT {X}"=w293:cdb[])  [unwired: 8 in, 1 out]
            n112 = Complex To Polar(r * e^(i*theta)=w293) -> (r=w292:dbl[])  [unwired: 1 out]
            n113 = Select(t=w315, s=w295, f=w316) -> (s? t:f=w314:i32)
            n114 = Array Subset "frequency of interest"(array=w292, index=w320, length=w314) -> (w291:dbl[])
            n115 = Array Max & Min(array=w291) -> (max value=w326:dbl, max index (indices)=w304:i32)  [unwired: 2 out]
            n116 = Greater?(x=w326, y=w317) -> (0:w310:bool)
            n117 = Not(x=w310) -> (.not. x?=w296:bool)
            n118 = feedback #5(40.0) -> (w319:dbl)
            n119 = case shown="True" w310 {
              tunnel: w304 -> [_ w328]
              tunnel: w320 -> [_ w329]
              tunnel: w311 -> [_ w330]
              tunnel: [w327 w331] -> w294
              tunnel: w319 -> [w327 _]
              frame False {
              }
              frame True {
                n120 = Add(x=w329, y=w328) -> (x+y=w332:i32)
                n121 = Multiply(x=w332, y=w330) -> (x*y=w331:dbl)
              }
            }
            n122 = feedback-in #5(w294) -> ()
          }
        }
        "Low-Energy Warning" <- w200
        n123 = call <vilib>:"High Resolution Relative Seconds.vi"() -> ("relative seconds"=w195:dbl)
      }
      frame #2 {
        n124 = call <vilib>:"High Resolution Relative Seconds.vi"() -> ("relative seconds"=w336:dbl)
      }
    }
    n125 = flat-sequence {
      tunnel: w114 -> [w341]
      tunnel: [w341] -> w176
      tunnel: [w345] -> w175
      tunnel: [w344] -> w174
      tunnel: w173 -> [w343]
      tunnel: [w339] -> w172
      tunnel: [w342] -> w128
      tunnel: w153 -> [w340]
      tunnel: [w340] -> w154
      tunnel: [w339] -> w150
      tunnel: w146 -> [w338]
      tunnel: w176 -> [w352]
      tunnel: [w353] -> w159
      tunnel: [w351] -> w163
      tunnel: w154 -> [w348]
      tunnel: w150 -> [w346]
      tunnel: w159 -> [w427]
      tunnel: [w427] -> w158
      tunnel: [w426] -> w157
      tunnel: w158 -> [w438]
      tunnel: w172 -> [w439]
      tunnel: w140 -> [w437]
      tunnel: [w438] -> w168
      tunnel: [w436] -> w167
      tunnel: [w435] -> w166
      tunnel: [w434] -> w162
      tunnel: [w431] -> w147
      tunnel: w148 -> [w430]
      tunnel: [w443] -> w142
      tunnel: [w444] -> w130
      tunnel: [w445] -> w178
      tunnel: w168 -> [w445]
      tunnel: w167 -> [w444]
      tunnel: w166 -> [w443]
      tunnel: [w442] -> w129
      frame #0 {
        n126 = call <vilib>:"High Resolution Relative Seconds.vi"() -> ("relative seconds"=w342:dbl)
        n127 = call "Sub_sample_unique_pin_locations.vi"("Modeling Parameters"=w341, "FEA Nodes"=w338, "Initial Pin Location"=w343) -> ("Unique Samples"=w339:i32[], "Sample PDF"=w345:dbl[], "Standard Deviation"=w344:dbl)  [unwired: 6 in]
      }
      frame #1 {
        n128 = call <vilib>:"High Resolution Relative Seconds.vi"() -> ("relative seconds"=w351:dbl)
        n129 = Array Size(array=w346) -> (size(s)=w347:i32)
        n130 = Not Equal To 0?(x="Eigenvalue Method") -> (x != 0?=w350:bool)
        n131 = case shown="True" w350 {
          tunnel: w346 -> [w356 w375]
          tunnel: [w355 w374] -> w353
          tunnel: w352 -> [_ w373]
          tunnel: w347 -> [w357 w372]
          tunnel: "Eigenvalue Method" -> [_ w371]
          tunnel: w348 -> [w354 _]
          frame False {
            n132 = for "For Loop: Worker Loop" {
              N: w357 -> [_]
              workers-P: w357 -> [_]
              tunnel: w356 -> [w360] mode=indexing
              tunnel: [w364] -> w355 mode=indexing
              tunnel: w354 -> [w359]
              (unwired) 3 ("Mode Count")
              n133 = Unbundle By Name(w359) -> ("LEMP"=w358:T12)
              n134 = Increment(x="Mode Count") -> (x+1=w361:i32)
              n135 = call "Sub_online_LEMP_Update_LabVIEW.vi"("Effected DOF"=w360, "Mode count"=w361, "LEMP"=w358) -> ("Updated Eigenvalues"=w363:dbl[])
              n136 = Complex To Re/Im ("Complex To Cartesian.vi")(x + iy=w363) -> (x=w370:dbl[])  [unwired: 1 out]
              n137 = Square Root ("Square Root.vi")(x=w370) -> (sqrt(x)=w369:dbl[])
              n138 = Divide(x=w369, y=6.283185307179586) -> (x/y=w365:dbl[])
              n139 = Sort 1D Array(array=w365) -> (sorted array=w367:dbl[])
              n140 = Index Array(array=w367, index=0) -> (element=w364:dbl)
            }
          }
          frame True {
            n141 = for "For Loop: Worker Loop" {
              N: w372 -> [_]
              tunnel: [w383] -> w374 mode=indexing
              tunnel: w375 -> [w380] mode=indexing
              tunnel: w373 -> [w376]
              workers-P: w372 -> [_]
              tunnel: w371 -> [w377]
              n142 = call "Sub_FEA_Make_M_and K_Matrices.vi"("Pin Location"=w380, "Modeling Parameters"=w376) -> ("K Matrix"=w379:dbl[][], "M Matrix"=w378:dbl[][])  [unwired: 8 in]
              n143 = case shown="\"2-LabVIEW M^-1K eigenvalues\"" w377 {
                tunnel: w378 -> [w392 w398 w406 _ _ _ _]
                tunnel: w379 -> [w391 w396 w408 _ _ _ _]
                tunnel: [w393 w401 w409 cdb[] [] ("Eigenvalues") cdb[] [] ("Eigenvalues") cdb[] [] ("Eigenvalues") cdb[] [] ("Eigenvalues")] -> w381
                frame "1-LabVIEW generalized eigenvalues", Default {
                  w394 = T13 0 items=["Eigenvalues", "Eigenvalues & Vectors"] ("output option")
                  n144 = call-poly <vilib>:"Array To Matrix.vi"("Real 2D Array"=w391) -> ("Real Matrix"=w390:T14)
                  n145 = call-poly <vilib>:"Array To Matrix.vi"("Real 2D Array"=w392) -> ("Real Matrix"=w389:T14)
                  n146 = call-poly <vilib>:"Generalized Eigenvalues and Vectors.vi"("output option"=w394, "B"=w389, "A"=w390) -> ("Eigenvalues"=w393:cdb[])  [unwired: 3 in, 2 out]
                }
                frame "2-LabVIEW M^-1K eigenvalues" {
                  w400 = T13 0 items=["Eigenvalues", "Eigenvalues & Vectors"] ("output option")
                  w403 = 0 items=["General", "Symmetric"] ("matrix type")
                  # "Inv(M)*K"
                  n147 = call-poly <vilib>:"Array To Matrix.vi"("Real 2D Array"=w398) -> ("Real Matrix"=w397:T14)
                  n148 = call-poly <vilib>:"Inverse Matrix.vi"("matrix type"=Matrix_Type_of_Inverse_Matrix."Positive Definite", "Input Matrix"=w397) -> ("Inverse Matrix"=w404:T14)  [unwired: 1 out]
                  n149 = call-poly <vilib>:"Array To Matrix.vi"("Real 2D Array"=w396) -> ("Real Matrix"=w395:T14)
                  n150 = call-poly <vilib>:"Multiply.vi"("Real Matrix B"=w395, "Real Matrix A"=w404) -> ("A * B"=w402:T14)
                  n151 = call-poly <vilib>:"Eigenvalues and Vectors.vi"("output option"=w400, "matrix type"=w403, "Input Matrix"=w402) -> ("Eigenvalues"=w401:cdb[])  [unwired: 2 out]
                }
                frame "3-LabVIEW Cholesky Factorization" {
                  w411 = T13 0 items=["Eigenvalues", "Eigenvalues & Vectors"] ("output option")
                  w412 = 1 items=["General", "Symmetric"] ("matrix type")
                  # "LabVIEW Cholesky"
                  n152 = call-poly <vilib>:"Array To Matrix.vi"("Real 2D Array"=w406) -> ("Real Matrix"=w405:T14)
                  n153 = call-poly <vilib>:"Cholesky Factorization.vi"("A"=w405) -> ("Cholesky"=w420:T14)  [unwired: 1 out]
                  n154 = Transpose Matrix(1:w420) -> (0:w421:T14)
                  n155 = call-poly <vilib>:"Inverse Matrix.vi"("Input Matrix"=w421) -> ("Inverse Matrix"=w419:T14)  [unwired: 1 in, 1 out]
                  n156 = call-poly <vilib>:"Array To Matrix.vi"("Real 2D Array"=w408) -> ("Real Matrix"=w407:T14)
                  n157 = call-poly <vilib>:"Multiply.vi"("Real Matrix B"=w407, "Real Matrix A"=w419) -> ("A * B"=w417:T14)
                  n158 = call-poly <vilib>:"Inverse Matrix.vi"("Input Matrix"=w420) -> ("Inverse Matrix"=w418:T14)  [unwired: 1 in, 1 out]
                  n159 = call-poly <vilib>:"Multiply.vi"("Real Matrix B"=w418, "Real Matrix A"=w417) -> ("A * B"=w416:T14)
                  n160 = Transpose Matrix(1:w416) -> (0:w415:T14)
                  n161 = call-poly <vilib>:"Add.vi"("Real Matrix B"=w415, "Real Matrix A"=w416) -> ("A + B"=w413:T14)
                  n162 = Divide(x=w413, y=2.0) -> (x/y=w410:T14)
                  n163 = call-poly <vilib>:"Eigenvalues and Vectors.vi"("output option"=w411, "matrix type"=w412, "Input Matrix"=w410) -> ("Eigenvalues"=w409:cdb[])  [unwired: 2 out]
                }
                frame "4-Cholesky Factorization CPU SGL" {
                }
                frame "5-Cholesky Factorization CPU FXP" {
                }
                frame "6-Cholesky Factorization FPGA SGL" {
                }
                frame "7-Cholesky Factorization FPGA SGL SCL" {
                }
              }
              n164 = Complex To Re/Im ("Complex To Cartesian.vi")(x + iy=w381) -> (x=w388:dbl[])  [unwired: 1 out]
              n165 = Square Root ("Square Root.vi")(x=w388) -> (sqrt(x)=w387:dbl[])
              n166 = Divide(x=w387, y=6.283185307179586) -> (x/y=w382:dbl[])
              n167 = Sort 1D Array(array=w382) -> (sorted array=w385:dbl[])
              n168 = Index Array(array=w385, index=0) -> (element=w383:dbl)
            }
          }
        }
      }
      frame #2 {
        n169 = call <vilib>:"High Resolution Relative Seconds.vi"() -> ("relative seconds"=w426:dbl)
      }
      frame #3 {
        n170 = Subtract(x=w437, y=w438) -> (x-y=w441:dbl[])
        n171 = Absolute Value(x=w441) -> (abs(x)=w433:dbl[])
        n172 = call <vilib>:"High Resolution Relative Seconds.vi"() -> ("relative seconds"=w434:dbl)
        n173 = Array Max & Min(array=w433) -> (min value=w429:dbl, min index (indices)=w440:i32)  [unwired: 2 out]
        n174 = Build Array (concatenate)(w430, w429) -> (w432:dbl[])
        n175 = call "Sub_truncate_buffer.vi"("array"=w432, "samples"=50) -> ("array"=w431:dbl[])  [unwired: 9 in]
        n176 = Index Array(array=w439, index=w440) -> (element=w436:i32)
        n177 = Index Array(array=w438, index=w440) -> (element=w435:dbl)
      }
      frame #4 {
        n178 = call <vilib>:"High Resolution Relative Seconds.vi"() -> ("relative seconds"=w442:dbl)
      }
    }
    n179 = Build Array (concatenate)(w141, w140) -> (w138:dbl[])
    n180 = Build Array (concatenate)(w144, w142) -> (w139:dbl[])
    n181 = Build Array (concatenate)(w135, w130) -> (w133:dbl[])
    n182 = Build Array (concatenate)(w136, w134) -> (w132:dbl[])
    n183 = case shown="True" "Real-Time plotting" {
      tunnel: w174 -> [_ w464]
      tunnel: w173 -> [_ w463]
      tunnel: w146 -> [_ w462]
      tunnel: w175 -> [_ w461]
      tunnel: w178 -> [_ w460]
      tunnel: w155 -> [_ _]
      tunnel: w115 -> [_ w459]
      tunnel: w140 -> [_ w457]
      tunnel: w145 -> [_ w458]
      tunnel: w139 -> [_ w447]
      tunnel: w138 -> [_ w454]
      tunnel: w133 -> [_ w446]
      tunnel: w132 -> [_ w450]
      frame False {
      }
      frame True {
        n184 = case shown="True" "PDF" {
          tunnel: w464 -> [_ w473]
          tunnel: w463 -> [_ w472]
          tunnel: w462 -> [_ w471]
          tunnel: w461 -> [_ w470]
          frame False {
            n185 = Wait (ms)(milliseconds to wait=u32 4) -> ()  [unwired: 1 out]
          }
          frame True {
            n186 = Bundle("nodes of interest"=w471, "Sample PDF"=w470) -> (→"Probability Density Function":T15)  [unwired: 1 in]
            n187 = control-ref of="Probability Density Function"() -> (w467:refnum<vi>)
            n188 = call-poly <vilib>:"Continuous Moments.vi"("std"=w473, "mean"=w472) -> ("variance"=w468:dbl, "mean"=w466:dbl)  [unwired: 7 in, 1 out]
            n189 = call "sub_plot_PDF_in_real_time.vi"("mean"=w466, "variance"=w468, "XYGraph in"=w467) -> ()  [unwired: 9 in]
          }
        }
        n190 = call "Convert to Dynamic Data"("Array"=w447) -> ("Dynamic Data Type"=w455:dynamicdata)  [unwired: 3 in]
        n191 = call "Convert to Dynamic Data2"("Array"=w454) -> ("Dynamic Data Type"=w453:dynamicdata)  [unwired: 3 in]
        n192 = call "Convert to Dynamic Data3"("Array"=w446) -> ("Dynamic Data Type"=w451:dynamicdata)  [unwired: 3 in]
        n193 = call "Convert to Dynamic Data4"("Array"=w450) -> ("Dynamic Data Type"=w449:dynamicdata)  [unwired: 3 in]
        n194 = Merge Signals(w455, w453) -> (→"Frequencies":dynamicdata)
        n195 = Merge Signals(w451, w449) -> (→"Position":dynamicdata)
        "FEA Frequencies" <- w460
        "Acceleration Data" <- w459
        "1st Nat. Freq. (Hz) 2" <- w457
        "FFT" <- w458
      }
    }
    n196 = call <vilib>:"High Resolution Relative Seconds.vi"() -> ("relative seconds"=w126:dbl)
    n197 = call "Sub_truncate_buffer.vi"("array"=w139, "samples"=w131) -> ("array"=w143:dbl[])  [unwired: 9 in]
    n198 = call "Sub_truncate_buffer.vi"("array"=w138, "samples"=w131) -> ("array"=w119:dbl[])  [unwired: 9 in]
    n199 = call "Sub_truncate_buffer.vi"("array"=w133, "samples"=w131) -> ("array"=w137:dbl[])  [unwired: 9 in]
    n200 = call "Sub_truncate_buffer.vi"("array"=w132, "samples"=w131) -> ("array"=w120:dbl[])  [unwired: 9 in]
    n201 = Subtract(x=w126, y=w128) -> (x-y=w127:dbl)
    n202 = Absolute Value(x=w127) -> (abs(x)=w125:dbl)
    n203 = Array Max & Min(array=w119) -> (max value=→"max value":dbl, min value=→"min value":dbl)  [unwired: 2 out]
    n204 = Multiply(x=w125, y=1000.0) -> (x*y=→"Cycle time (ms)":dbl)
  }
  n205 = disable-structure shown="Disabled" {
    frame Disabled {
      n206 = call-poly <vilib>:"DAQmx Write.vi"("data"=bool[] [FALSE, FALSE]) -> ("task/channels in"=w474:refnum<k21>, "task out"=w476:refnum<k21>, "error out"=w475:errorcluster)  [unwired: 11 in, 1 out]
      n207 = call <vilib>:"DAQmx Clear Task.vi"("task in"=w476, "error in"=w475) -> ()  [unwired: 13 in, 1 out]
    }
    frame Enabled {
    }
  }
  n208 = call "Sub_time_constant_start_2022.vi"("time_frequency_calculations_start"=w69, "time_accelerometer_acquire_start"=w66, "Experimental Results IN"=w63, "time_subsample_start"=w68, "time_FEA_end"=w65, "time_frequency_calculations_end"=w70, "time_compare_start"=w71, "measured_pin_location_tt"=w31, "time_cycle_end"=w67, "time_cycle_start"=w72, "time_FEA_start"=w36) -> ("Experimental Results OUT"=w47:T8)  [unwired: 8 in]
  n209 = Unbundle By Name(w47) -> ("time_average_cycle"=w18:dbl)
  n210 = Unbundle By Name(w61) -> ("beam_length"=w60:dbl, "number_of_FEA_nodes"=w62:i32)
  n211 = Decrement(x=w62) -> (x-1=w59:i32)
  n212 = Format Date/Time String() -> (date/time string=w75:string)  [unwired: 3 in]
  n213 = Divide(x=w60, y=w59) -> (x/y=w58:dbl)
  n214 = Multiply(x=w35, y=w58) -> (x*y=w19:dbl[])
  n215 = Bundle By Name("Y"=w21, "dt"=w18) -> (w46:waveform(dbl))  [unwired: 1 in]
  n216 = Bundle By Name("Y"=w34, "dt"=w18) -> (w45:waveform(dbl))  [unwired: 1 in]
  n217 = Bundle By Name("Y"=w20, "dt"=w18) -> (w24:waveform(dbl))  [unwired: 1 in]
  n218 = Bundle By Name("Y"=w19, "dt"=w18) -> (w23:waveform(dbl))  [unwired: 1 in]
  n219 = Multiply(x=1000.0, y=w18) -> (x*y=→"average cycle time (ms)":dbl)
  n220 = Build Array(w46, w45) -> (→"1st Nat. Freq. (Hz) 4":waveform(dbl)[])
  n221 = Build Array(w24, w23) -> (→"1st Nat. Freq. (Hz) 5":waveform(dbl)[])
  n222 = Bundle By Name(cluster=w47, "measured_frequency"=w21, "date_time"=w75, "estimated_pin_node"=w35, "estimated_frequency"=w34, "estimated_pin_location"=w19, "measured_pin_location"=w20) -> (w50:T8)
  n223 = case shown="True" "Save Acceleration Data" {
    tunnel: [w478 w485] -> w49
    tunnel: w50 -> [w478 w484]
    tunnel: w48 -> [_ w483]
    tunnel: w33 -> [_ _]
    tunnel: w32 -> [_ _]
    frame False {
    }
    frame True {
      n224 = Unbundle By Name(w484) -> ("accelerometer_sample_rate"=w479:dbl)
      n225 = Reciprocal(x=w479) -> (1/x=w480:dbl)
      n226 = Array Size(array=w483) -> (size(s)=w481:i32)
      n227 = for {
        N: w481 -> [_]
        tunnel: w480 -> [w487]
        tunnel: [w486] -> w482 mode=indexing
        i -> [w488]
        n228 = Multiply(x=w487, y=w488) -> (x*y=w486:dbl)
      }
      n229 = Bundle By Name(cluster=w484, "time_acceleration_data"=w482, "acceleration_data"=w483) -> (w485:T8)
    }
  }
  n230 = flat-sequence {
    tunnel: w61 -> [w518]
    tunnel: w49 -> [w514]
    tunnel: "file name" -> [w509]
    tunnel: [w507] -> w57
    frame #0 {
      n231 = Unbundle(w514) -> ("time_average_cycle"=w519:dbl, "measured_frequency"=w520:dbl[], "date_time"=w521:string, "estimated_pin_node"=w522:i32[], "time_cycle_start"=w523:dbl[], "measured_pin_location"=w524:dbl[], "estimated_frequency"=w525:dbl[], "acceleration_data"=w526:dbl[], "accelerometer_sample_rate"=w527:dbl, "displacement_sample_rate"=w528:dbl, "time_compare_start"=w529:dbl[], "time_subsample_start"=w530:dbl[], "time_FEA_start"=w531:dbl[], "time_FEA_end"=w532:dbl[], "time_cycle_end"=w533:dbl[], "time_accelerometer_aquire_start"=w534:dbl[], "time_frequency_calculations_start"=w535:dbl[], "time_frequency_calculations_end"=w536:dbl[], "measured_pin_location_tt"=w517:dbl[], "time_ACC_data_collection_start"=w516:dbl, "time_acceleration_data"=w515:dbl[], "estimated_pin_location"=w508:dbl[], "scaling_factor_Hz_per_pin_to_frequency_resolution"=w506:dbl, "Std_Dev_equale_particles_divided_3"=w505:bool, "Auto_FFT_length"=w504:bool, "windowed_acc_data"=w503:dbl[][], "FFT"=w502:dbl[][])
      n232 = Unbundle(w518) -> ("beam_length"=w501:dbl, "youngs_modulus"=w500:dbl, "torsion_spring"=w499:dbl, "beam_height"=w498:dbl, "beam_width"=w497:dbl, "beam_density"=w496:dbl, "number_of_FEA_nodes"=w495:i32, "FFT_data_length"=w494:i32, "standard_deviation"=w493:dbl, "number_of_particles"=w492:i32, "min_FFT_power_value"=w491:dbl, "initial_pin_node"=w490:i32, "accelerometer_mass"=w489:dbl)  [unwired: 5 out]
      n233 = Number To Decimal String(number=w509) -> (decimal integer string=w510:string)  [unwired: 1 in]
      n234 = Current VI's Path() -> (path=w539:path)
      n235 = Strip Path(path=w539) -> (stripped path=w538:path)  [unwired: 1 out]
      n236 = Concatenate Strings("data\\data_" ("name or relative path"), w510, ".json" ("name or relative path")) -> (w511:string)
      n237 = Bundle("time_average_cycle"=w519, "measured_frequency"=w520, "date_time"=w521, "estimated_pin_node"=w522, "time_cycle_start"=w523, "measured_pin_location"=w524, "estimated_frequency"=w525, "acceleration_data"=w526, "accelerometer_sample_rate"=w527, "displacement_sample_rate"=w528, "time_compare_start"=w529, "time_subsample_start"=w530, "time_FEA_start"=w531, "time_FEA_end"=w532, "time_cycle_end"=w533, "time_accelerometer_aquire_start"=w534, "time_frequency_calculations_start"=w535, "time_frequency_calculations_end"=w536, "measured_pin_location_tt"=w517, "time_ACC_data_collection_start"=w516, "time_acceleration_data"=w515, "estimated_pin_location"=w508, "scaling_factor_Hz_per_pin_to_frequency_resolution"=w506, "Std_Dev_equale_particles_divided_3"=w505, "Auto_FFT_length"=w504, "windowed_acc_data"=w503, "FFT"=w502, "beam_length"=w501, "youngs_modulus"=w500, "torsion_spring"=w499, "beam_height"=w498, "beam_width"=w497, "beam_density"=w496, "number_of_FEA_nodes"=w495, "FFT_data_length"=w494, "standard_deviation"=w493, "number_of_particles"=w492, "min_FFT_power_value"=w491, "initial_pin_node"=w490, "accelerometer_mass"=w489) -> (w507:T16)  [unwired: 1 in]
      n238 = Build Path(base path=w538, name or relative path=w511) -> (appended path=w537:path)
      n239 = Flatten To JSON(anything=w507) -> (JSON string=w540:string)  [unwired: 2 in, 1 out]
      n240 = Write to Text File(file (use dialog)=w537, text=w540) -> (refnum out=w542:refnum<file>, error out=w541:errorcluster)  [unwired: 2 in, 1 out]
      n241 = Close File(refnum=w542, error in=w541) -> ()  [unwired: 2 out]
    }
  }
  n242 = flat-sequence {
    tunnel: w57 -> [w547]
    frame #0 {
      n243 = Unbundle By Name(w547) -> ("measured_pin_location_tt"=w558:dbl[], "measured_pin_location"=w546:dbl[], "time_cycle_end"=w557:dbl[], "estimated_pin_location"=w545:dbl[])
      n244 = Unbundle By Name(w547) -> ("measured_pin_location_tt"=w556:dbl[], "measured_pin_location"=w552:dbl[], "time_acceleration_data"=w543:dbl[], "acceleration_data"=w554:dbl[])
      n245 = Bundle("measured_pin_location_tt"=w558, "measured_pin_location"=w546) -> (w559:T17)  [unwired: 1 in]
      n246 = Bundle("time_acceleration_data"=w543, "acceleration_data"=w554) -> (w553:T18)  [unwired: 1 in]
      n247 = Multiply(x=w552, y=100.0 ("x")) -> (x*y=w549:dbl[])
      n248 = Bundle("time_cycle_end"=w557, "estimated_pin_location"=w545) -> (w544:T19)  [unwired: 1 in]
      n249 = Subtract(x=w549, y=6.8) -> (x-y=w548:dbl[])
      n250 = Bundle("measured_pin_location_tt"=w556, w548) -> (w555:cluster{"measured_pin_location_tt":dbl[], dbl[]})  [unwired: 1 in]
      n251 = Build Array(w555, w553) -> ()  [unwired: 1 out]
      n252 = Build Array(w559, w544) -> ()  [unwired: 1 out]
    }
  }
